vi "hse-application_SetFpgaVersion.vi"(8 "error in":errorcluster, 11 "FPGA Version Number":string) -> (0 "error out":errorcluster)   [LabVIEW 2022 SP3, in "hse-application.lvclass"]
doc: "Stores the version number of the FPGA bitfile (if any) for later usage (display, logging, ...).\n\n\n\n____\nHAMPEL SOFTWARE ENGINEERING v3.8.0 (2023-12-18 14:41)"
uses:
  hse-application.lvclass
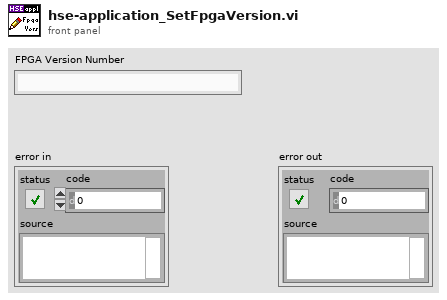
[diagram p1: front panel]
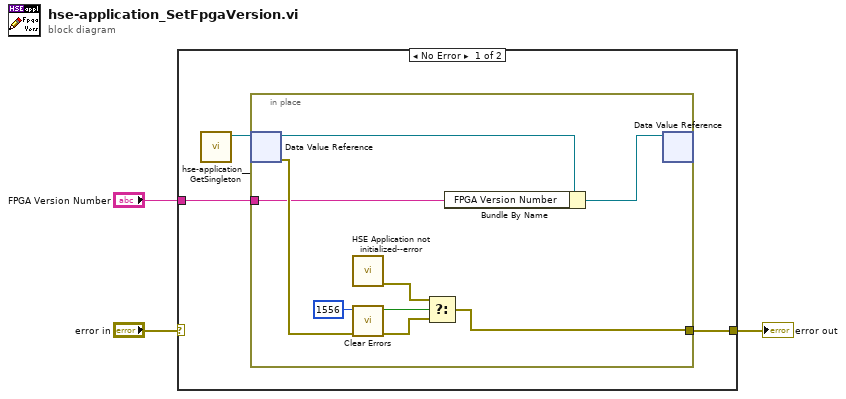
[diagram p0: block diagram]
diagram:
  n1 = case shown="No Error" "error in" {
    selector: "error in" -> [_ w16]
    tunnel: [w6 w16] -> w2
    tunnel: "FPGA Version Number" -> [w4 _]
    frame No Error {
      n2 = call "hse-application__GetSingleton.vi"() -> ("ApplicationClass DVR"=w5:refnum<data-value>)  [unwired: 10 in, 1 out]
      n3 = in-place "In Place Element Structure" {
        in-place-border: [w12] -> w6
        in-place-border: w4 -> [w10]
        n4 = in-place-dvr #1(w5) -> (w11:refnum<class "hse-application.lvclass">, w13:errorcluster)
        n5 = call "HSE Application not initialized--error.vi"() -> ("error out"=w15:errorcluster)  [unwired: 11 in]
        n6 = call <vilib>:"Clear Errors.vi"("error in (no error)"=w13, "specific error code to clear (0: all)"=1556) -> ("error out"=w14:errorcluster, "specific error cleared?"=w7:bool)  [unwired: 4 in]
        n7 = Select(t=w15, s=w7, f=w14) -> (s? t:f=w12:errorcluster)
        n8 = Bundle By Name(cluster=w11, "FPGA Version Number"=w10) -> (w9:refnum<class "hse-application.lvclass">)
        n9 = in-place-dvr #1(w9) -> ()  [unwired: 2 out]
      }
    }
    frame Error {
    }
  }
  "error out" <- w2
